vi "manual_setRefractiveIndex.vi"(8 "error":errorcluster, 9 "rindex":dbl format="%#_13g", 10 "axis":i32, 11 "connection ID":refnum<k5>) -> (0 "error out":errorcluster, 2 "axis_out":i32, 3 "connection ID out":refnum<k5>)   [LabVIEW 2016, in "sen_api.lvlib"]
doc: "Sets the manually configured refractive index for the compensation mode 2. The input range is defined to be greater than 1."
uses:
  sen_api.lvlib
panel:
  out "jsonRespIn":string
  out "JSON-response":string="{\"jsonrpc\":\"2.0\",\"method\":\"\",\"params\":[5,1.245,true,\"name\"],\"id\":\"1\"}"
  out "JSON request":string
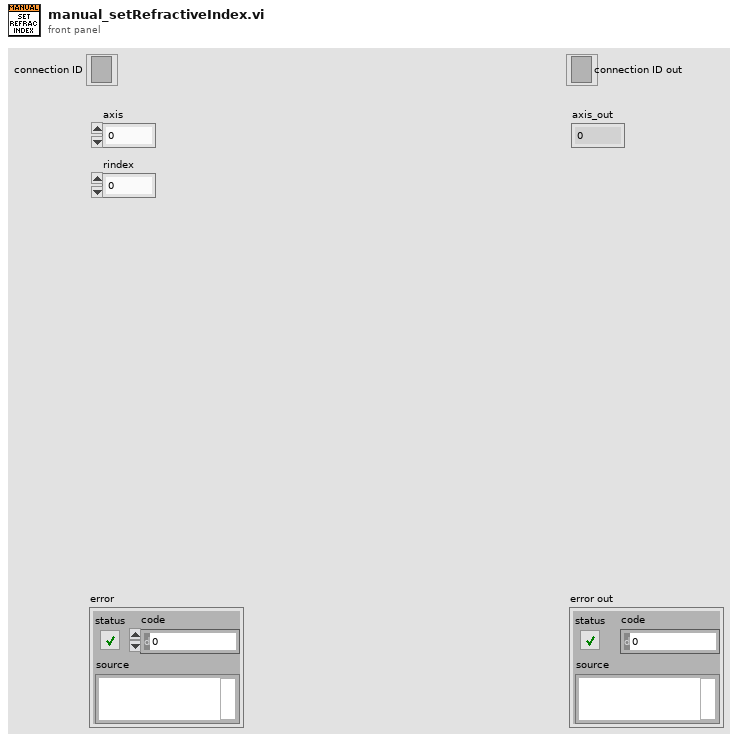
[diagram p1: front panel]
types:
  T1 = cluster{"jsonrpc":string, "method":string, "params":string[], "id":string, "api":i32, "pid":string}
  T2 = enum16{"Standard", "Buffered", "CRLF", "Immediate"}
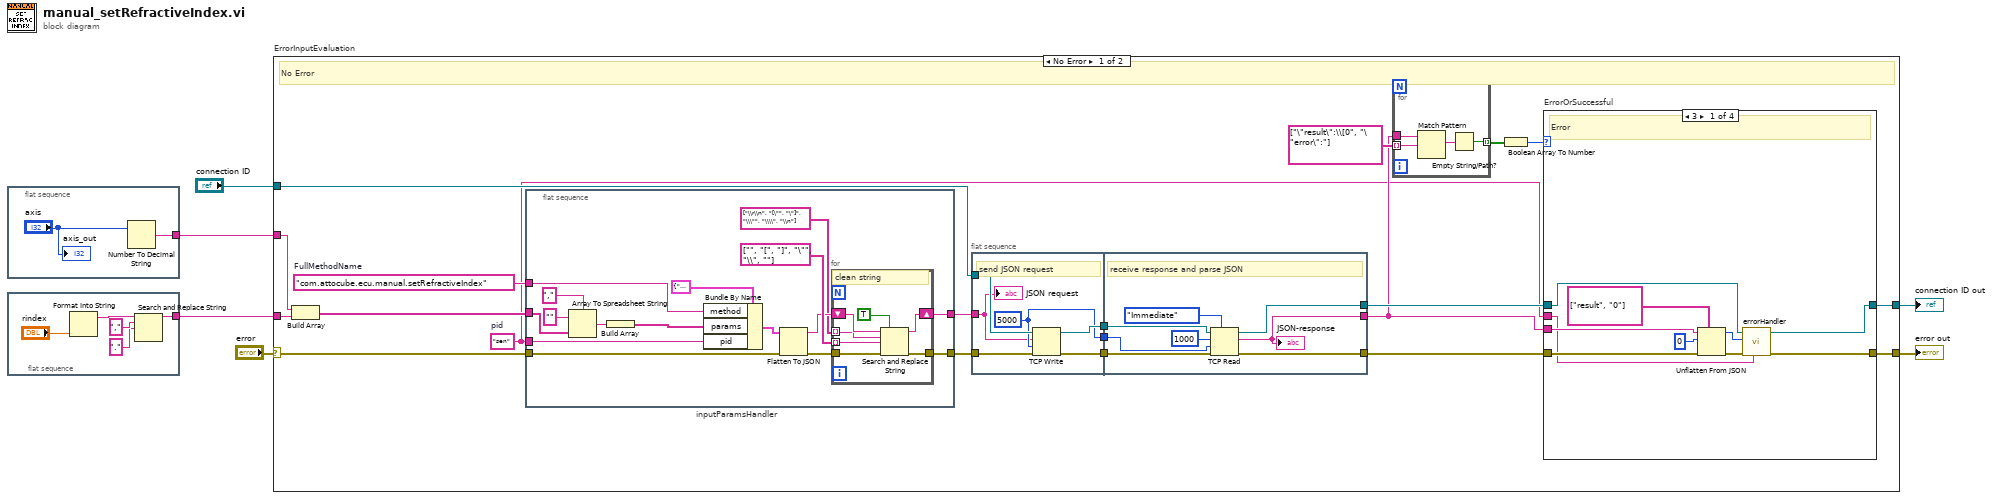
[diagram p0: block diagram]
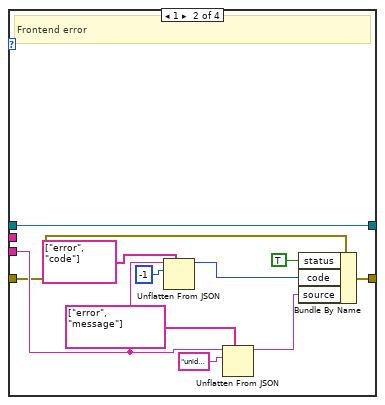
[diagram p2: hidden frame]
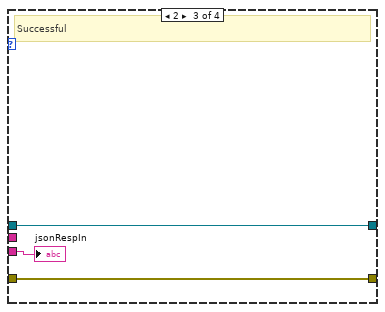
[diagram p3: hidden frame]
diagram:
  n1 = flat-sequence "in_axis" {
    tunnel: [w8] -> w2
    frame #0 {
      n2 = Number To Decimal String(number="axis") -> (decimal integer string=w8:string)  [unwired: 1 in]
      "axis_out" <- "axis"
    }
  }
  n3 = flat-sequence "in_double" {
    tunnel: [w9] -> w1
    frame #0 {
      n4 = Format Into String("rindex") -> (resulting string=w12:string)  [unwired: 3 in, 1 out]
      n5 = Search and Replace String(input string=w12, search string=",", replace string="." ("search string")) -> (result string=w9:string)  [unwired: 5 in, 3 out]
    }
  }
  n6 = case "ErrorInputEvaluation" shown="No Error" "error" {
    selector: "error" -> [w20 w101]
    tunnel: "connection ID" -> [w30 w102]
    tunnel: [w22 w101] -> w5
    tunnel: [w23 w102] -> w4
    tunnel: w2 -> [w15 _]
    tunnel: w1 -> [w14 _]
    frame No Error {
      w16 = "sen"  # pid
      w21 = "com.attocube.ecu.manual.setRefractiveIndex"  # FullMethodName
      # "No Error"
      n7 = Build Array ("ParametersArrayString")(w15, w14) -> (w19:string[])
      n8 = flat-sequence "inputParamsHandler" {
        tunnel: [w37] -> w18
        tunnel: w19 -> [w44]
        tunnel: w20 -> [w42]
        tunnel: [w39] -> w17
        tunnel: w21 -> [w45]
        tunnel: w16 -> [w34]
        frame #0 {
          n9 = Array To Spreadsheet String(delimiter (Tab)=",", array=w44, 3:"" ("format string")) -> (spreadsheet string=w47:string)
          n10 = Build Array "Build Array"(w47) -> (w43:string[])
          n11 = Bundle By Name(cluster=T1 {"jsonrpc"="2.0", "method"="com.attocube.amc.res.setRESReadOutFreq", "params"=[], "id"="1", "api"=2, "pid"=""}, "method"=w45, "params"=w43, "pid"=w34) -> (w46:T1)
          n12 = Flatten To JSON(anything=w46, error in (no error)=w42) -> (JSON string=w38:string, 11:w40:errorcluster)  [unwired: 1 in]
          n13 = for {
            tunnel: string[] ["\\r\\n", "[\"", "\"]", "\\\"", "\\\\", "\\n"] ("search string") -> [w53] mode=indexing
            tunnel: string[] ["", "[", "]", "\"", "\\", ""] ("replace string (\"\")") -> [w52] mode=indexing
            shift-right: [w55] -> w37
            shift-left: w38 -> [w54]
            tunnel: w40 -> [w51]
            tunnel: [w50] -> w39
            # "clean string"
            n14 = Search and Replace String(replace all?=TRUE ("replace all? (F)"), input string=w54, search string=w53, replace string=w52, error in=w51) -> (result string=w55:string, error out=w50:errorcluster)  [unwired: 3 in, 2 out]
          }
        }
      }
      n15 = flat-sequence {
        tunnel: w30 -> [w92]
        tunnel: [w90] -> w33
        tunnel: [w91] -> w32
        tunnel: w17 -> [w87]
        tunnel: [w89] -> w31
        tunnel: w18 -> [w88]
        tunnel: [w96] -> w26
        tunnel: w33 -> [w98]
        tunnel: w32 -> [w97]
        tunnel: [w94] -> w25
        tunnel: w31 -> [w95]
        tunnel: [w93] -> w24
        frame #0 {
          w89 = 5000 ("timeout ms (25000)")
          # "send JSON request"
          n16 = TCP Write(connection ID=w92, data in=w88, error in (no error)=w87, 9:w89) -> (connection ID out=w90:refnum<k5>, error out=w91:errorcluster)  [unwired: 1 out]
          "JSON request" <- w88
        }
        frame #1 {
          # "receive response and parse JSON"
          n17 = TCP Read(connection ID=w98, bytes to read=1000, error in (no error)=w97, 7:T2."Immediate" ("mode (standard)"), 9:w95) -> (connection ID out=w96:refnum<k5>, data out=w93:string, error out=w94:errorcluster)
          "JSON-response" <- w93
        }
      }
      n18 = for {
        tunnel: string[] ["\"result\":\\[0", "\"error\":"] ("path") -> [w59] mode=indexing
        tunnel: [w57] -> w28 mode=indexing
        tunnel: w24 -> [w60]
        n19 = Match Pattern(string=w60, regular expression=w59) -> (match substring=w58:string)  [unwired: 1 in, 3 out]
        n20 = Empty String/Path?(string/path=w58) -> (empty?=w57:bool)
      }
      n21 = Boolean Array To Number(Boolean array=w28) -> (number=w27:u32)
      n22 = case "ErrorOrSuccessful" shown="3" w27 {
        tunnel: w24 -> [w64 w73 w82 _]
        tunnel: w26 -> [w68 w71 w84 w86]
        tunnel: [w66 w71 w84 w86] -> w23
        tunnel: [w67 w74 w83 w85] -> w22
        tunnel: w25 -> [w70 w72 w83 w85]
        tunnel: w16 -> [w61 _ _ _]
        frame 3 {
          # "Error"
          n23 = Unflatten From JSON(path=string[] ["result", "0"], JSON string=w64, type and defaults=0, error in (no error)=w70) -> (value=w62:i32, error out=w69:errorcluster)  [unwired: 3 in]
          n24 = call "errorHandler.vi"("pid"=w61, "error in"=w69, "errNbr"=w62, "connection ID"=w68) -> ("error out 2"=w67:errorcluster, "connection ID out"=w66:refnum<k5>)  [unwired: 6 in]
        }
        frame 1 {
          # "Frontend error"
          n25 = Unflatten From JSON(path=string[] ["error", "code"], JSON string=w73, type and defaults=-1) -> (value=w80:i32)  [unwired: 4 in, 1 out]
          n26 = Unflatten From JSON(path=string[] ["error", "message"], JSON string=w73, type and defaults="unidentified error") -> (value=w81:string)  [unwired: 4 in, 1 out]
          n27 = Bundle By Name(cluster=w72, "status"=TRUE, "code"=w80, "source"=w81) -> (w74:errorcluster)
        }
        frame 2 {
          # "Successful"
          "jsonRespIn" <- w82
        }
        frame Default {
          # "NoResponse"
        }
      }
    }
    frame Error {
      # "Error"
    }
  }
  "error out" <- w5
  "connection ID out" <- w4
